vi "Notifier AE.vi"(7 "Cmd":string, 8 "error in (no error)":errorcluster, 10 "String":string) -> (0 "error out":errorcluster)   [LabVIEW 2013, in "main.lvlib"]
uses:
  main.lvlib
  Load.vi
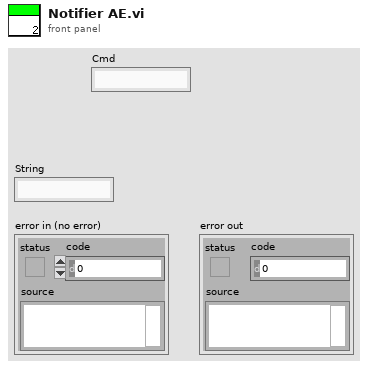
[diagram p1: front panel]
types:
  T1 = enum32{"Invalid", "Standard", "Closed", "Hidden", "Minimized", "Maximized"}
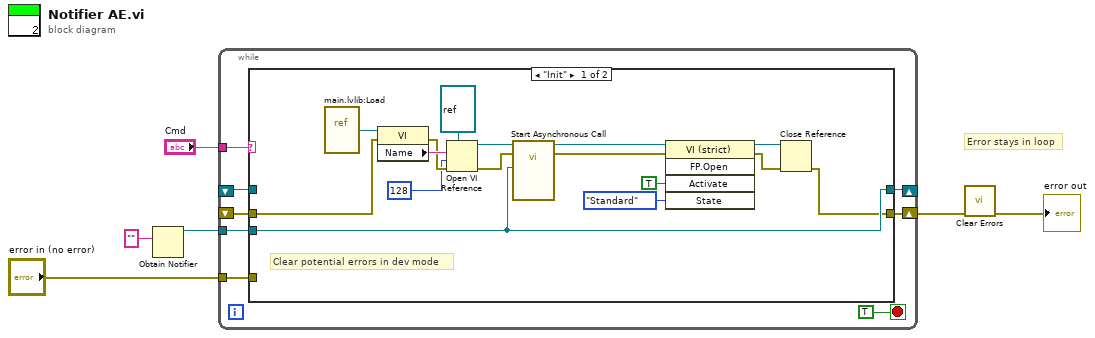
[diagram p0: block diagram]
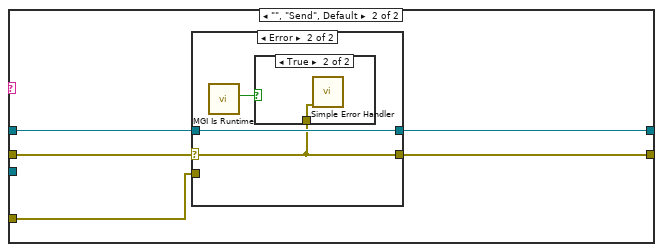
[diagram p2: hidden frame]
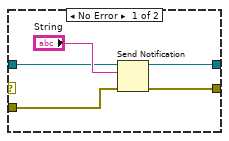
[diagram p3: hidden frame]
diagram:
  # "Error stays in loop"
  n1 = Obtain Notifier(notification data type="") -> (notifier out=w4:refnum<notifier>)  [unwired: 3 in, 2 out]
  n2 = while {
    tunnel: "Cmd" -> [w12]
    shift-right: [w11] -> _
    shift-left: _ -> [w10]
    tunnel: w4 -> [w9]
    shift-right: [w8] -> w3
    shift-left: _ -> [w14]
    tunnel: "error in (no error)" -> [w7]
    stop <- TRUE stop-if-true
    n3 = case shown="\"Init\"" w12 {
      tunnel: w14 -> [w15 w32]
      tunnel: [w24 w35] -> w11
      tunnel: w10 -> [_ w34]
      tunnel: w9 -> [w24 _]
      tunnel: [w16 w33] -> w8
      tunnel: w7 -> [_ w31]
      frame "Init" {
        # "Clear potential errors in dev mode"
        n4 = vi-ref "main.lvlib:Load.vi"() -> (w30:refnum<vi>)
        n5 = property class="VI"(reference=w30, error in=w15) -> (error out=w25:errorcluster, "Name"=w29:string)  [unwired: 1 out]
        n6 = Open VI Reference(type specifier VI Refnum (for type only)=refnum<vi> refnum, vi path=w29, options=128, error in (no error)=w25) -> (vi reference=w27:refnum<vi>, error out=w26:errorcluster)  [unwired: 2 in]
        n7 = call-by-ref "Start Asynchronous Call"(reference=w27, error in=w26, "notifier out"=w24) -> (reference out=w23:refnum<vi>, error out=w20:errorcluster)  [unwired: 11 in]
        n8 = invoke class="VI (strict)" method="FP.Open"(reference=w23, error in=w20, "Activate"=TRUE ("Activate?"), "State"=T1."Standard") -> (reference out=w19:refnum<vi>, error out=w18:errorcluster)  [unwired: 1 in, 3 out]
        n9 = Close Reference(reference=w19, error in (no error)=w18) -> (error out=w16:errorcluster)
      }
      frame "", "Send", Default {
        n10 = case shown="Error" w32 {
          selector: w32 -> [_ w41]
          tunnel: [w39 w43] -> w35
          tunnel: w34 -> [w38 w43]
          tunnel: [w37 w41] -> w33
          tunnel: w31 -> [w36 _]
          frame No Error {
            n11 = Send Notification(notification="String", notifier=w38, error in (no error)=w36) -> (notifier out=w39:refnum<notifier>, error out=w37:errorcluster)
          }
          frame Error {
            n12 = call <userlib>:"MGI Is Runtime.vi"() -> ("Run Time System?"=w42:bool)  [unwired: 7 in]
            n13 = case shown="True" w42 {
              tunnel: w41 -> [_ w44]
              frame False {
              }
              frame True {
                n14 = call <vilib>:"Simple Error Handler.vi"("error in (no error)"=w44) -> ()  [unwired: 4 in, 5 out]
              }
            }
          }
        }
      }
    }
  }
  n15 = call <vilib>:"Clear Errors.vi"("error in (no error)"=w3) -> ("error out"=→"error out":errorcluster)  [unwired: 6 in]
